vi "Set Axis Speed.vi"(8 "error in (no error)":errorcluster, 10 "Axis":string, 11 "Stage Actor.lvlib:Stage.lvclass":refnum<class "Stage.lvclass">) -> (0 "error out":errorcluster, 3 "Actor out":refnum<class "Actor.lvclass">)   [LabVIEW 2018, in "Stage Actor.lvlib" / "Stage.lvclass"]
uses:
  Stage.lvclass
  <vilib>/ActorFramework/Actor/Actor.lvclass
  C:/Program Files (x86)/National Instruments/LabVIEW 2018/vi.lib/ActorFramework/Actor/Actor.lvclass
  Stage.lvclass/Stage.ctl
  <instrlib>/Zaber A Series/Zaber A Series.lvlib
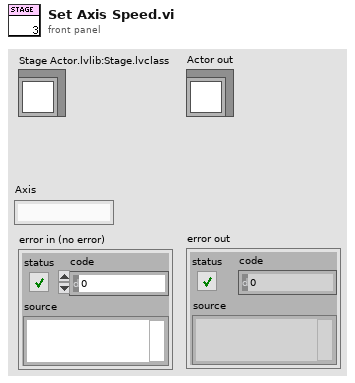
[diagram p1: front panel]
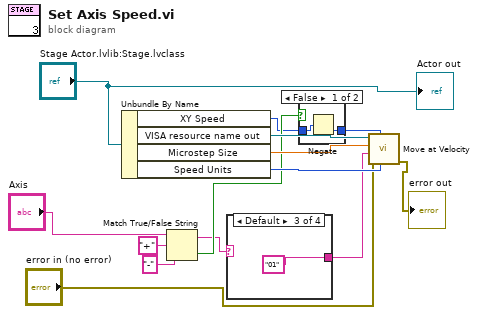
[diagram p0: block diagram]
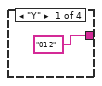
[diagram p2: hidden frame]
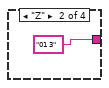
[diagram p3: hidden frame]
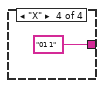
[diagram p4: hidden frame]
diagram:
  n1 = Unbundle By Name("Stage Actor.lvlib:Stage.lvclass") -> ("XY Speed"=w6:i16, "VISA resource name out"=w14:refnum<visa-resource-name>, "Microstep Size"=w11:dbl, "Speed Units"=w12:u16)
  n2 = Match True/False String(2:"-" ("false string"), 3:"+" ("true string"), 4:"Axis") -> (0:w7:bool, 1:w4:string)
  n3 = case shown="Default" w4 {
    tunnel: ["01 2" "01 3" "01" "01 1"] -> w3
    frame "Y" {
    }
    frame "Z" {
    }
    frame Default {
    }
    frame "X" {
    }
  }
  n4 = case shown="False" w7 {
    tunnel: w6 -> [w20 w21]
    tunnel: [w19 w21] -> w5
    frame False {
      n5 = Negate(x=w20) -> (-x=w19:i16)
    }
    frame True {
    }
  }
  n6 = call <instrlib>:"Move at Velocity.vi"("Units (0: device speed units)"=w12, "Velocity"=w5, "error in (no error)"="error in (no error)", "Device and Axis"=w3, "Microstep Size (0)"=w11, "VISA resource name"=w14) -> ("error out"=→"error out":errorcluster)  [unwired: 4 in, 1 out]
  "Actor out" <- "Stage Actor.lvlib:Stage.lvclass"
